vi "TCP_Init.vi"(8 "error in (no error)":errorcluster, 9 "timeout ms (60000)":i32, 10 "remote port or service name":u16, 11 "address":string) -> (0 "error out 2":errorcluster, 3 "ID OUT":refnum<k5>, 4 "State":bool=TRUE)   [LabVIEW 2022 SP3]
panel:
  # "192.168.127.200\n5025"
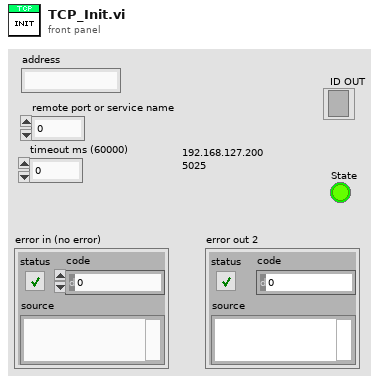
[diagram p1: front panel]
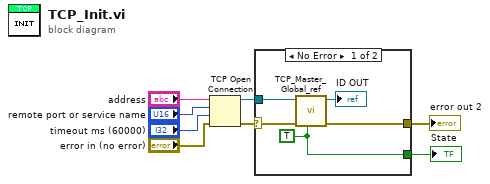
[diagram p0: block diagram]
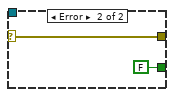
[diagram p2: hidden frame]
diagram:
  n1 = TCP Open Connection(address="address", remote port or service name="remote port or service name", timeout ms (60000)="timeout ms (60000)", error in (no error)="error in (no error)") -> (connection ID=w8:refnum<k5>, error out=w3:errorcluster)  [unwired: 1 in]
  n2 = case shown="No Error" w3 {
    selector: w3 -> [w12 w15]
    tunnel: w8 -> [w13 _]
    tunnel: [w10 w15] -> w2
    tunnel: [w9 FALSE ("Read:F/Wirte:T")] -> w1
    frame No Error {
      w9 = TRUE ("Read:F/Wirte:T")
      n3 = call "TCP_Master_Global_ref.vi"("Read:F/Wirte:T"=w9, "error in (no error) 2"=w12, "ID IN"=w13) -> ("error out 2"=w10:errorcluster, "ID OUT"=→"ID OUT":refnum<k5>)  [unwired: 7 in]
    }
    frame Error {
    }
  }
  "error out 2" <- w2
  "State" <- w1
